vi "Decision_Timer.vi"(8 "error in":errorcluster, 10 "Time has Elapsed":bool, 11 "Last State":T1) -> (0 "error out":errorcluster, 3 "State":T1)   [LabVIEW 2023]
uses:
  Controls/State.ctl
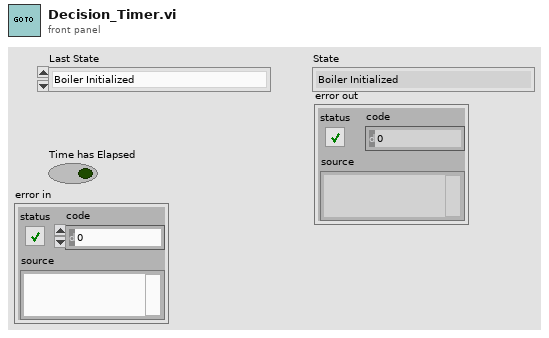
[diagram p1: front panel]
types:
  T1 = typedef "State.ctl" = enum16{"Boiler Initialized", "Boiler Ready", "Start Pre-Purge", "Pre-Purge Complete", "Pilot On", "Pilot Proved", "Force Draft Fan ON", "Boiler Running", "Start Shutdown Purge", "Shutdown Purge Complete", "Wait for Something"}
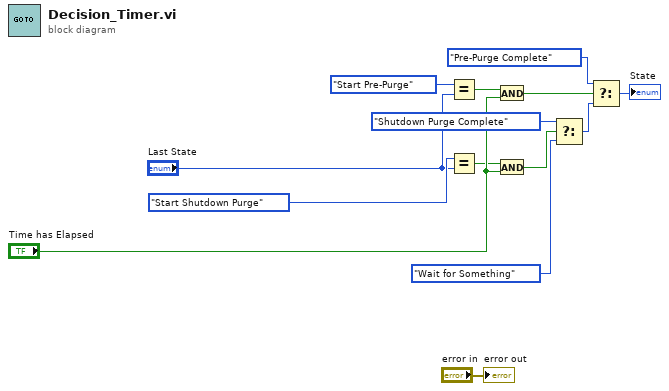
[diagram p0: block diagram]
diagram:
  n1 = Equal?(x=State."Start Pre-Purge", y="Last State") -> (x = y?=w6:bool)
  n2 = Equal?(x=State."Start Shutdown Purge", y="Last State") -> (x = y?=w10:bool)
  n3 = And(x=w6, y="Time has Elapsed") -> (x .and. y?=w5:bool)
  n4 = And(x=w10, y="Time has Elapsed") -> (x .and. y?=w12:bool)
  n5 = Select(t=State."Shutdown Purge Complete", s=w12, f=State."Wait for Something") -> (s? t:f=w7:T1)
  n6 = Select(t=State."Pre-Purge Complete", s=w5, f=w7) -> (s? t:f=→"State":T1)
  "error out" <- "error in"
